vi "CRYFlatten Curve Library.vi"(11 "CurLibData":T1 {"Waveforms"."Y dB ref" format="%.1f"; "Waveforms"."Y axis" items=["Log", "Lin"]; "Waveforms"."Y data" items=["dB", "Lin"]; "Waveforms"."X data" items=["dB", "Lin"]; "Values"."Z data" items=["dB", "Lin"]; "Values"."X data" items=["dB", "Lin"]; "Values"."Y data" items=["dB", "Lin"]; "Values"."Z dB ref" format="%.1f"; "Values"."Z axis" items=["Log", "Lin"]; "Values"."X dB ref" format="%.1f"; "Values"."X axis" items=["Log", "Lin"]; "Values"."Y axis" items=["Log", "Lin"]; "Values"."Y dB ref" format="%.1f"; "Values"."Curve"."z" format="%.2f"; "Values"."Curve"."y" format="%.2f"; "Values"."Curve"."x" format="%.2f"; "Results"."Margin" format="%.2f"; "Curves"."Z data" items=["dB", "Lin"]; "Curves"."X data" items=["dB", "Lin"]; "Curves"."Y data" items=["dB", "Lin"]; "Curves"."Z dB ref" format="%.1f"; "Curves"."Z axis" items=["Log", "Lin"]; "Curves"."X dB ref" format="%.1f"; "Curves"."X axis" items=["Log", "Lin"]; "Curves"."Y axis" items=["Log", "Lin"]; "Curves"."Y dB ref" format="%.1f"; "Curves"."Curve"."z" format="%.2f"; "Curves"."Curve"."y" format="%.2f"; "Curves"."Curve"."x" format="%.2f"}) -> (3 "CurLib flattened":string)   [LabVIEW 2013]
uses:
  Control/CRYCurve Library Cluster.ctl
  CRYSystem/Typedef Control/CRYData Cluster Array.ctl
  CRYSystem/Typedef Control/CRYData Cluster.ctl
  CRYSystem/Typedef Control/CRYResult Cluster Array.ctl
  CRYSystem/Typedef Control/CRYResult Cluster.ctl
  CRYSystem/Typedef Control/CRYWaveform Cluster Array.ctl
  CRYSystem/Typedef Control/CRYWaveform Cluster.ctl
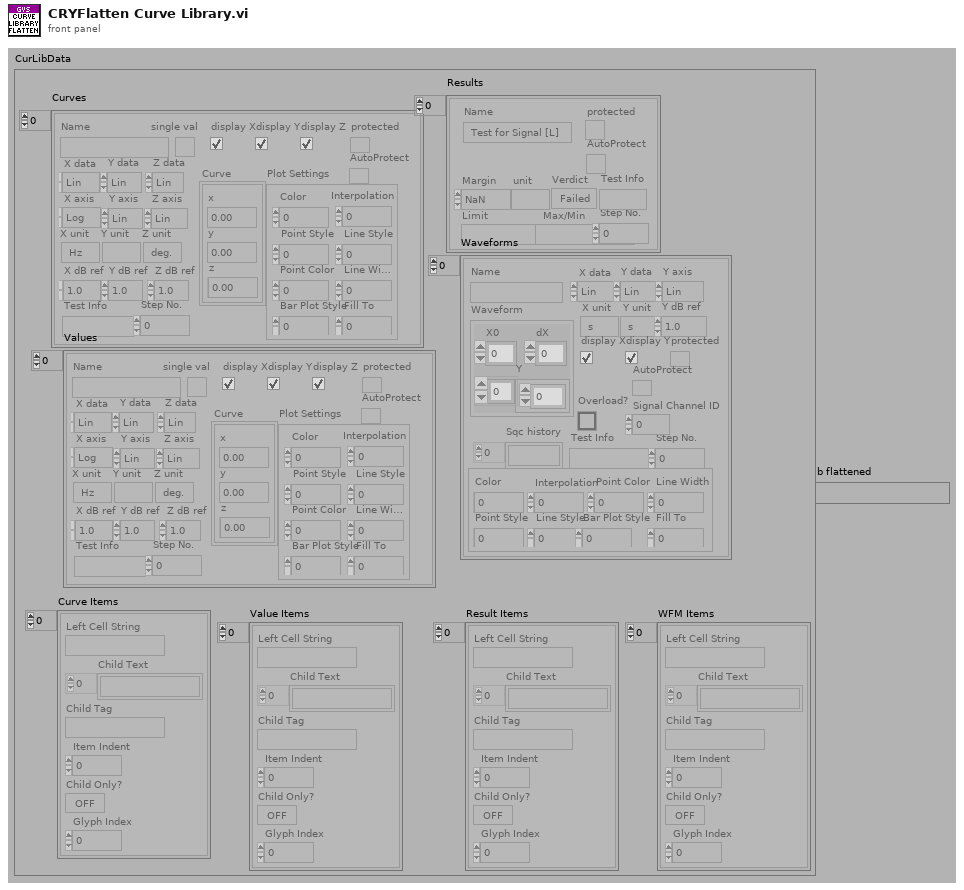
[diagram p1: front panel]
types:
  T1 = typedef "CRYCurve Library Cluster.ctl" = cluster{"Curves":T2, "Results":T4, "Values":T2, "Waveforms":T6, "Curve Items":cluster{"Left Cell String":string, "Child Text":string[], "Child Tag":string, "Item Indent":i32, "Child Only?":bool, "Glyph Index":i32}[], "Value Items":cluster{"Left Cell String":string, "Child Text":string[], "Child Tag":string, "Item Indent":i32, "Child Only?":bool, "Glyph Index":i32}[], "Result Items":cluster{"Left Cell String":string, "Child Text":string[], "Child Tag":string, "Item Indent":i32, "Child Only?":bool, "Glyph Index":i32}[], "WFM Items":cluster{"Left Cell String":string, "Child Text":string[], "Child Tag":string, "Item Indent":i32, "Child Only?":bool, "Glyph Index":i32}[]}
  T2 = typedef "CRYData Cluster Array.ctl" = T3[]
  T3 = typedef "CRYData Cluster.ctl" = cluster{"Name":string, "Curve":cluster{"x":dbl, "y":dbl, "z":dbl}[], "X data":u16, "Y data":u16, "Z data":u16, "X axis":u16, "Y axis":u16, "Z axis":u16, "X unit":string, "Y unit":string, "Z unit":string, "X dB ref":dbl, "Y dB ref":dbl, "Z dB ref":dbl, "single val":bool, "protected":bool, "display X":bool, "display Y":bool, "display Z":bool, "Test Info":string, "Step No.":i32, "Plot Settings":cluster{"Color":u32, "Interpolation":u8, "Point Style":u8, "Line Style":u8, "Point Color":u32, "Line Width":u8, "Bar Plot Style":u8, "Fill To":i16}, "AutoProtect":bool}
  T4 = typedef "CRYResult Cluster Array.ctl" = T5[]
  T5 = typedef "CRYResult Cluster.ctl" = cluster{"Name":string, "Margin":dbl, "unit":string, "Verdict":bool, "Limit":string, "Max/Min":string, "protected":bool, "Step No.":i32, "Test Info":string, "AutoProtect":bool}
  T6 = typedef "CRYWaveform Cluster Array.ctl" = T7[]
  T7 = typedef "CRYWaveform Cluster.ctl" = cluster{"Waveform":cluster{"X0":dbl, "dX":dbl, "Y":sgl[]}, "X data":u16, "Y data":u16, "Y axis":u16, "X unit":string, "Y unit":string, "Y dB ref":dbl, "display Y":bool, "display X":bool, "Overload?":bool, "Test Info":string, "Step No.":i32, "Name":string, "protected":bool, "Sqc history":string[], "Signal Channel ID":i32, "Plot Settings":cluster{"Color":u32, "Interpolation":u8, "Point Style":u8, "Line Style":u8, "Point Color":u32, "Line Width":u8, "Bar Plot Style":u8, "Fill To":i16}, "AutoProtect":bool}
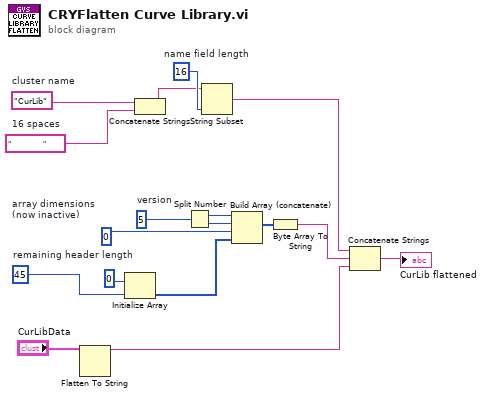
[diagram p0: block diagram]
diagram:
  w3 = u8 0  # array dimensions (now inactive)
  w6 = 16  # name field length
  w7 = "                "  # 16 spaces
  w8 = "CurLib"  # cluster name
  w13 = 45  # remaining header length
  w17 = u16 5  # version
  n1 = Flatten To String(anything="CurLibData") -> (data string=w2:string)  [unwired: 1 in, 4 out]
  n2 = Initialize Array(u8 0, w13) -> (w9:u8[])
  n3 = Concatenate Strings(w8, w7) -> (w5:string)
  n4 = Split Number(x=w17) -> (hi(x)=w16:u8, lo(x)=w15:u8)
  n5 = String Subset(string=w5, length (rest)=w6) -> (substring=w4:string)  [unwired: 1 out]
  n6 = Build Array (concatenate)(w16, w15, w3, w9) -> (w12:u8[])
  n7 = Byte Array To String(unsigned byte array=w12) -> (string=w10:string)
  n8 = Concatenate Strings(w4, w10, w2) -> (→"CurLib flattened":string)
